vi "update_jk.vi"(6 "J Output":dbl[](array[numeric]), 9 "Delta K":dbl, 10 "Learning Parameter":dbl, 11 "Weight":dbl[][](array[numeric])) -> (3 "Updated Weights":dbl[](array[numeric]))   [LabVIEW 2018]
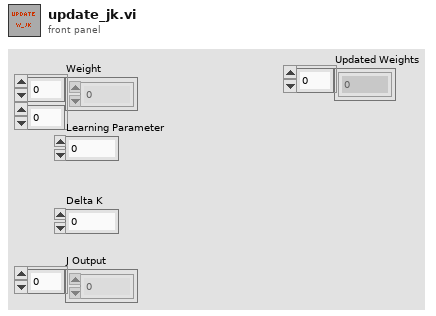
[diagram p1: front panel]
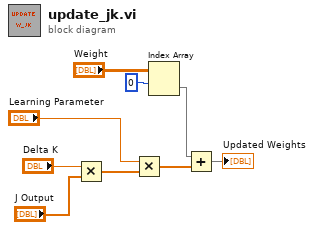
[diagram p0: block diagram]
diagram:
  n1 = Multiply(x="Delta K", y="J Output") -> (x*y=w7:dbl[])
  n2 = Multiply(x="Learning Parameter", y=w7) -> (x*y=w2:dbl[])
  n3 = Index Array(array="Weight", index (row)=0) -> (element=w3:dbl[])  [unwired: 1 in]
  n4 = Add(x=w3, y=w2) -> (x+y=→"Updated Weights":dbl[])
